vi "CarWash.vi"() -> ()   [LabVIEW 2023]
panel:
  in  "Tab Control":enum32{"Page 1", "Page 2"}(tab)
  in  "Refresh Button 2":bool
  out "String":string
  in  "Refresh Button":bool
  in  "Password":string
  in  "Username":string
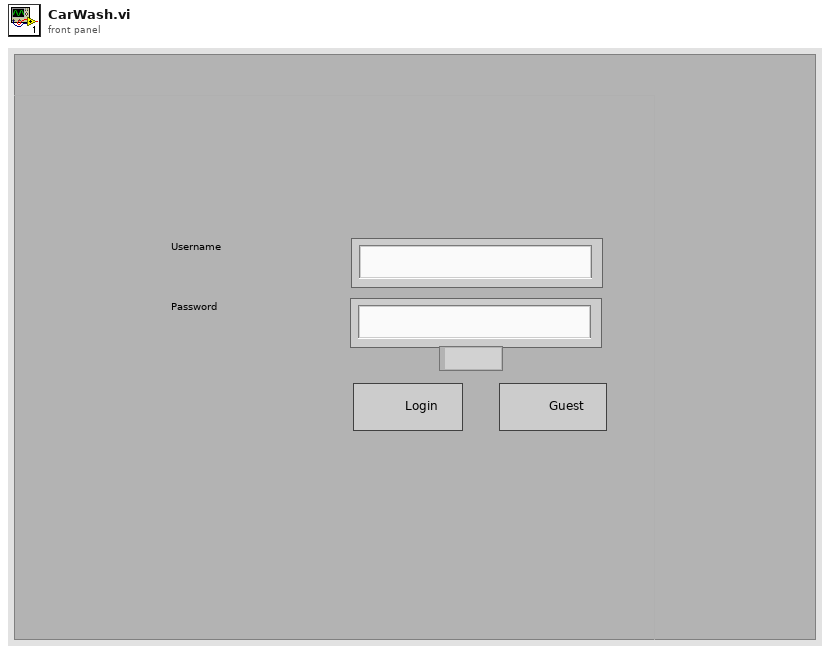
[diagram p1: front panel]
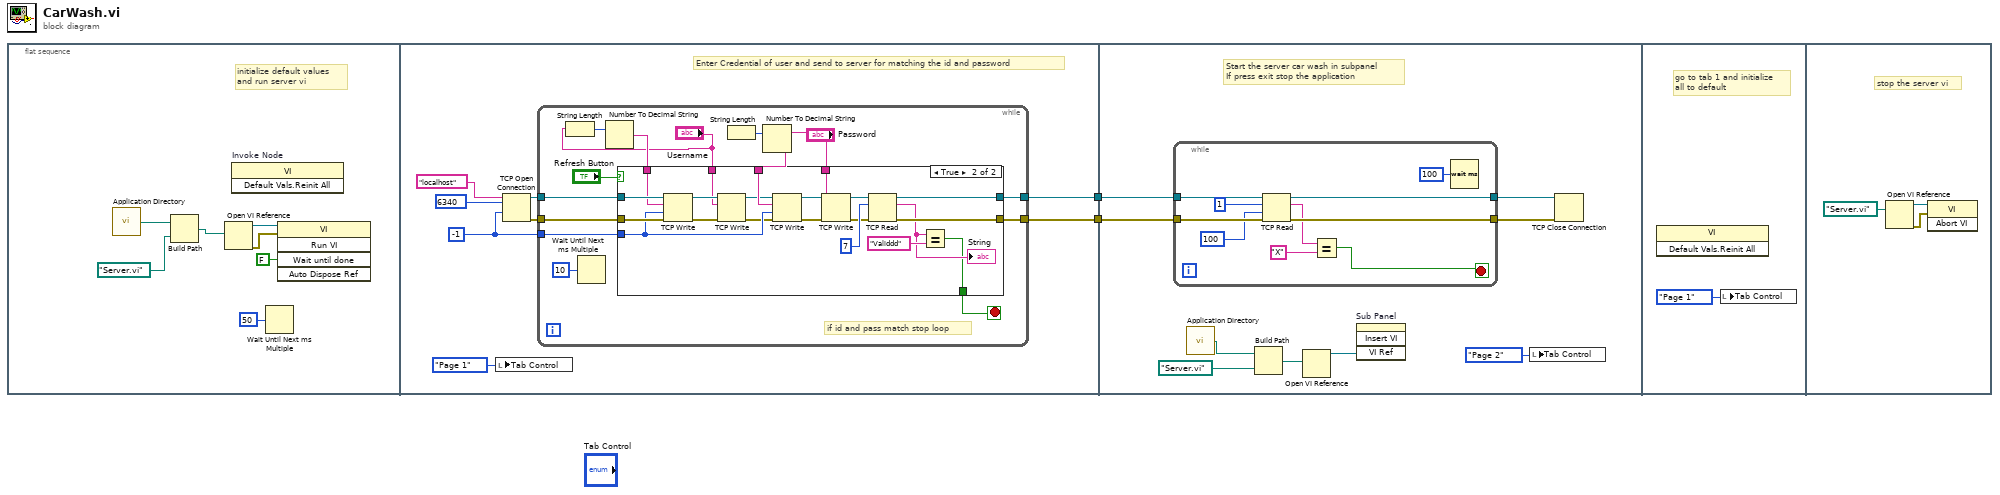
[diagram p0: block diagram]
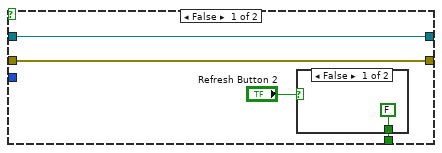
[diagram p2: hidden frame]
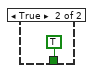
[diagram p3: hidden frame]
diagram:
  n1 = flat-sequence {
    tunnel: [w12] -> w2
    tunnel: [w11] -> w1
    tunnel: w2 -> [w63]
    tunnel: w1 -> [w62]
    frame #0 {
      # "initialize default values\nand run server vi"
      n2 = call <vilib>:"Application Directory.vi"() -> ("Application Directory"=w3:path)
      n3 = Build Path(base path=w3, name or relative path=path "Server.vi" ("vi path 2")) -> (appended path=w4:path)
      n4 = Open VI Reference(vi path=w4) -> (vi reference=w9:refnum<vi>, error out=w8:errorcluster)  [unwired: 5 in]
      n5 = invoke on="Invoke Node" class="VI" method="Default Vals.Reinit All"() -> ()  [unwired: 3 in, 3 out]
      n6 = Wait Until Next ms Multiple(millisecond multiple=u32 50) -> ()  [unwired: 1 out]
      n7 = invoke class="VI" method="Run VI"(reference=w9, error in=w8, "Wait until done"=FALSE ("Wait Until Done")) -> ()  [unwired: 2 in, 5 out]
    }
    frame #1 {
      w13 = -1 ("timeout ms (60000)")
      # "Enter Credential of user and send to server for matching the id and password"
      n8 = local write "Tab Control"(enum32{"Page 1", "Page 2"}."Page 1" ("Tab Control")) -> ()
      n9 = TCP Open Connection(address="localhost", remote port or service name=u16 6340, timeout ms (60000)=w13) -> (connection ID=w17:refnum<k5>, error out=w16:errorcluster)  [unwired: 2 in]
      n10 = while {
        tunnel: w13 -> [w27]
        tunnel: w17 -> [w29]
        tunnel: [w26] -> w12
        tunnel: w16 -> [w28]
        tunnel: [w25] -> w11
        stop <- w24 stop-if-true
        # "if id and pass match stop loop"
        n11 = String Length(string="Username") -> (length=w23:i32)
        n12 = Wait Until Next ms Multiple(millisecond multiple=u32 10 ("milliseconds to wait")) -> ()  [unwired: 1 out]
        n13 = Number To Decimal String(number=w23) -> (decimal integer string=w22:string)  [unwired: 1 in]
        n14 = String Length(string="Password") -> (length=w20:i32)
        n15 = Number To Decimal String(number=w20) -> (decimal integer string=w18:string)  [unwired: 1 in]
        n16 = case shown="True" "Refresh Button" {
          tunnel: w29 -> [w35 w58]
          tunnel: w28 -> [w34 w57]
          tunnel: w22 -> [_ w56]
          tunnel: w18 -> [_ w55]
          tunnel: w27 -> [_ w54]
          tunnel: [w35 w52] -> w26
          tunnel: [w34 w53] -> w25
          tunnel: [w33 w49] -> w24
          tunnel: "Username" -> [_ w43]
          tunnel: "Password" -> [_ w38]
          frame False {
            n17 = case shown="False" "Refresh Button 2" {
              tunnel: [FALSE TRUE] -> w33
              frame False {
              }
              frame True {
              }
            }
          }
          frame True {
            n18 = TCP Write(connection ID=w58, data in=w56, error in (no error)=w57, 9:w54) -> (connection ID out=w47:refnum<k5>, error out=w46:errorcluster)  [unwired: 1 out]
            n19 = TCP Write(connection ID=w47, data in=w43, error in (no error)=w46) -> (connection ID out=w44:refnum<k5>, error out=w45:errorcluster)  [unwired: 1 in, 1 out]
            n20 = TCP Write(connection ID=w44, data in=w55, error in (no error)=w45, 9:w54) -> (connection ID out=w40:refnum<k5>, error out=w39:errorcluster)  [unwired: 1 out]
            n21 = TCP Write(connection ID=w40, data in=w38, error in (no error)=w39) -> (connection ID out=w42:refnum<k5>, error out=w41:errorcluster)  [unwired: 1 in, 1 out]
            n22 = TCP Read(connection ID=w42, bytes to read=7, error in (no error)=w41) -> (connection ID out=w52:refnum<k5>, data out=w50:string, error out=w53:errorcluster)  [unwired: 2 in]
            "String" <- w50
            n23 = Equal?(x=w50, y="Validdd") -> (x = y?=w49:bool)
          }
        }
      }
    }
    frame #2 {
      # "Start the server car wash in subpanel\nIf press exit stop the application"
      n24 = while {
        tunnel: w63 -> [w76]
        tunnel: w62 -> [w75]
        tunnel: [w73] -> w61
        tunnel: [w72] -> w60
        stop <- w68 stop-if-true
        n25 = TCP Read(connection ID=w76, bytes to read=1, error in (no error)=w75, 9:100 ("timeout ms (25000)")) -> (connection ID out=w72:refnum<k5>, data out=w71:string, error out=w73:errorcluster)  [unwired: 1 in]
        n26 = Equal?(x=w71, y="X") -> (x = y?=w68:bool)
        n27 = Wait (ms)(milliseconds to wait=u32 100) -> ()  [unwired: 1 out]
      }
      n28 = call <vilib>:"Application Directory.vi"() -> ("Application Directory"=w65:path)
      n29 = Build Path(base path=w65, name or relative path=path "Server.vi" ("vi path 2")) -> (appended path=w67:path)
      n30 = Open VI Reference(vi path=w67) -> (vi reference=w66:refnum<vi>)  [unwired: 5 in, 1 out]
      n31 = invoke on="Sub Panel" class="SubPnl" method="Insert VI"("VI Ref"=w66) -> ()  [unwired: 3 in, 4 out]
      n32 = local write "Tab Control"(enum32{"Page 1", "Page 2"}."Page 2" ("Tab Control")) -> ()
      n33 = TCP Close Connection(connection ID=w60, error in (no error)=w61) -> ()  [unwired: 1 in, 2 out]
    }
    frame #3 {
      # "go to tab 1 and initialize\nall to default"
      n34 = invoke class="VI" method="Default Vals.Reinit All"() -> ()  [unwired: 3 in, 3 out]
      n35 = local write "Tab Control"(enum32{"Page 1", "Page 2"}."Page 1" ("Tab Control")) -> ()
    }
    frame #4 {
      # "stop the server vi"
      n36 = Open VI Reference(vi path=path "Server.vi" ("vi path 2")) -> (vi reference=w80:refnum<vi>, error out=w81:errorcluster)  [unwired: 5 in]
      n37 = invoke class="VI" method="Abort VI"(reference=w80, error in=w81) -> ()  [unwired: 1 in, 3 out]
    }
  }
